vi "TCP 서버.vi"() -> ()   [LabVIEW 2018]
uses:
  <vilib>/Analysis/NI_AALBase.lvlib
panel:
  in  "정지":bool
  out "웨이브폼 그래프":dbl[](graph)
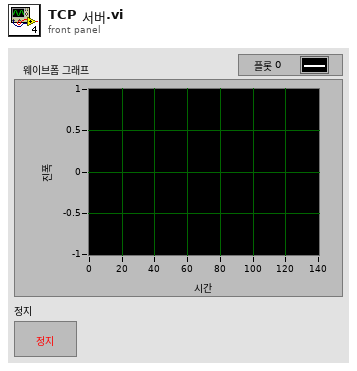
[diagram p1: front panel]
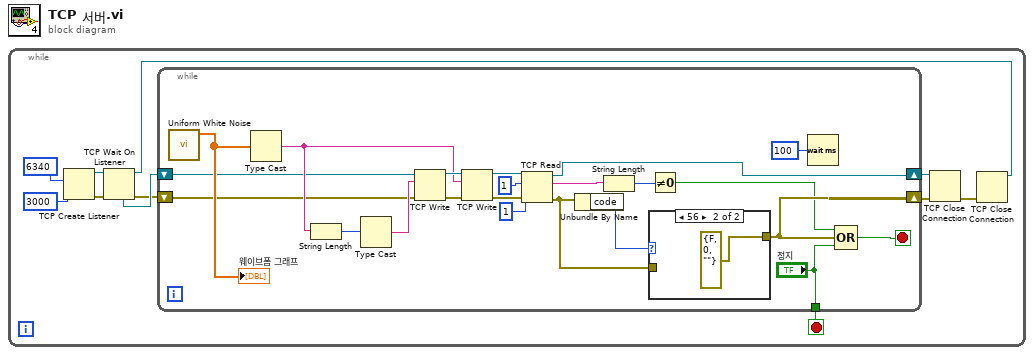
[diagram p0: block diagram]
diagram:
  n1 = while {
    stop <- w1 stop-if-true
    n2 = TCP Create Listener(9:3000 ("타임아웃 ms (25000)"), 10:u16 6340 ("포트")) -> (0:w8:errorcluster, 3:w11:refnum<k5>)  [unwired: 3 in, 1 out]
    n3 = TCP Wait On Listener(8:w8, 11:w11) -> (0:w3:errorcluster, 3:w6:refnum<k5>, 4:w5:refnum<k5>)  [unwired: 2 in, 2 out]
    n4 = while {
      shift-right: [w19] -> w4
      shift-left: w5 -> [w20]
      shift-right: [w14] -> w2
      shift-left: w3 -> [w18]
      tunnel: ["정지"] -> w1
      stop <- w15 stop-if-true
      n5 = call <vilib>:"Uniform White Noise.vi"() -> ("uniform white noise"=w28:dbl[])  [unwired: 10 in, 1 out]
      "웨이브폼 그래프" <- w28
      n6 = Type Cast(x=w28) -> (*(type *) &x=w27:string)  [unwired: 1 in]
      n7 = String Length(string=w27) -> (length=w26:i32)
      n8 = Type Cast(x=w26) -> (*(type *) &x=w25:string)  [unwired: 1 in]
      n9 = TCP Write(connection ID=w20, data in=w25, error in (no error)=w18) -> (connection ID out=w30:refnum<k5>, error out=w29:errorcluster)  [unwired: 1 in, 1 out]
      n10 = TCP Write(connection ID=w30, data in=w27, error in (no error)=w29) -> (connection ID out=w31:refnum<k5>, error out=w32:errorcluster)  [unwired: 1 in, 1 out]
      n11 = TCP Read(connection ID=w31, bytes to read=1 ("읽을 바이트"), error in (no error)=w32, 9:1 ("타임아웃 ms (25000)")) -> (connection ID out=w19:refnum<k5>, data out=w22:string, error out=w16:errorcluster)  [unwired: 1 in]
      n12 = Unbundle By Name(w16) -> ("code"=w17:i32)
      n13 = String Length(string=w22) -> (length=w21:i32)
      n14 = case shown="56" w17 {
        tunnel: w16 -> [w34 _]
        tunnel: [w34 errorcluster {"status"=FALSE, "code"=0, "source"=""} ("에러 상수")] -> w14
        frame Default {
        }
        frame 56 {
        }
      }
      n15 = Not Equal To 0?(x=w21) -> (x != 0?=w13:bool)
      n16 = Wait (ms)(milliseconds to wait=u32 100 ("대기 시간 (ms)")) -> ()  [unwired: 1 out]
      n17 = Compound Arithmetic op=OR(w13, w14, "정지") -> (w15:bool)
    }
    n18 = TCP Close Connection(connection ID=w4, error in (no error)=w2) -> (error out=w7:errorcluster)  [unwired: 1 in, 1 out]
    n19 = TCP Close Connection(connection ID=w6, error in (no error)=w7) -> ()  [unwired: 1 in, 2 out]
  }
